vi "Update Files for Review.vi"(8 "error in":errorcluster, 11 "Peer Review":refnum<class "Peer Review.lvclass">) -> (0 "error out":errorcluster)   [LabVIEW 2020, in "Peer Review.lvclass"]
uses:
  Peer Review.lvclass
  Peer Review.lvclass/Peer Review.ctl
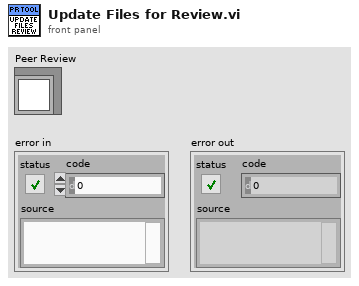
[diagram p1: front panel]
types:
  T1 = typedef "Peer Review.lvclass/File Info.ctl" = cluster{"File ID":i32, "Commit ID":i32, "Reviewed Hash":string, "Relative Path":string, "File Path":path, "File Checksum":string, "State":T2, "FP Changes":i32, "BD Changes":i32, "FP Bounds Error":dbl, "BD Bounds Error":dbl, "Lines Added":i32, "Lines Removed":i32, "Analysis Passes":i32, "Analysis Fails":i32, "Attribute Changes":i32, "Reentrancy State":string, "Cyclomatic Complexity":i32, "Node Count":i32, "Revision Number":u32, "LabVIEW Version":string, "Description":string, "Master Path":path, "Master Checksum":string, "VI Type":T3, "LabVIEW File":bool, "Review Complete":bool, "File Ref":refnum<vi>, "Master Revision":u32}
  T2 = typedef "Peer Review.lvclass/File State.ctl" = enum16{"Interrogation Needed", "Modified", "Deleted", "Added", "Matches Previous", "No Changes", "Moved", "Empty File"}
  T3 = typedef "Peer Review.lvclass/VI Type.ctl" = enum32{"invalid VI type", "Standard VI", "Control VI", "Global VI", "Polymorphic VI", "Configuration VI", "SubSystem", "Facade VI", "Method VI", "Statechart Diagram VI"}
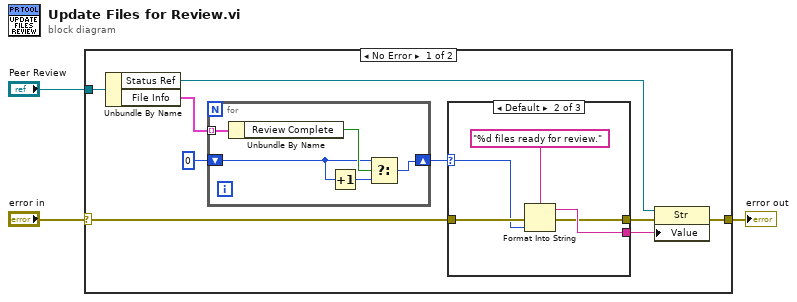
[diagram p0: block diagram]
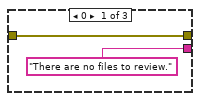
[diagram p2: hidden frame]
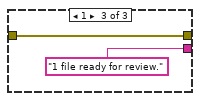
[diagram p3: hidden frame]
diagram:
  n1 = case shown="No Error" "error in" {
    selector: "error in" -> [w10 w27]
    tunnel: "Peer Review" -> [w9 _]
    tunnel: [w8 w27] -> w1
    frame No Error {
      n2 = Unbundle By Name(w9) -> ("Status Ref"=w7:refnum<vi>, "File Info"=w5:T1[])
      n3 = for {
        tunnel: w5 -> [w17] mode=indexing
        shift-right: [w13] -> w4
        shift-left: 0 -> [w14]
        n4 = Unbundle By Name(w17) -> ("Review Complete"=w16:bool)
        n5 = Increment(x=w14) -> (x+1=w15:i32)
        n6 = Select(t=w14, s=w16, f=w15) -> (s? t:f=w13:i32)
      }
      n7 = case shown="Default" w4 {
        selector: w4 -> [_ w20 _]
        tunnel: ["There are no files to review." ("t") w23 "1 file ready for review." ("Value")] -> w12
        tunnel: w10 -> [w18 w22 w25]
        tunnel: [w18 w21 w25] -> w11
        frame 0 {
        }
        frame Default {
          n8 = Format Into String(format string="%d files ready for review." ("Value"), error in=w22, w20) -> (resulting string=w23:string, error out=w21:errorcluster)  [unwired: 1 in]
        }
        frame 1 {
        }
      }
      n9 = property on="Property Node" class="Str"(reference=w7, error in=w11, "Value"=w12) -> (error out=w8:errorcluster)  [unwired: 1 out]
    }
    frame Error {
    }
  }
  "error out" <- w1
